vi "Update Expression.vi"(8 "error in (no error)":errorcluster, 10 "Expression":string, 11 "Cron in":refnum<class "Cron.lvclass">) -> (0 "error out":errorcluster, 1 "updated":bool, 3 "Cron out":refnum<class "Cron.lvclass">)   [LabVIEW 2013, in "openCron.lvlib" / "Cron.lvclass"]
uses:
  Cron.lvclass
  Cron.lvclass/Cron.ctl
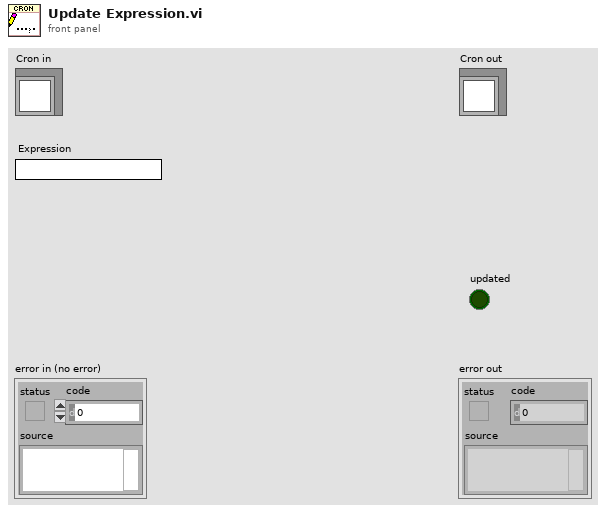
[diagram p1: front panel]
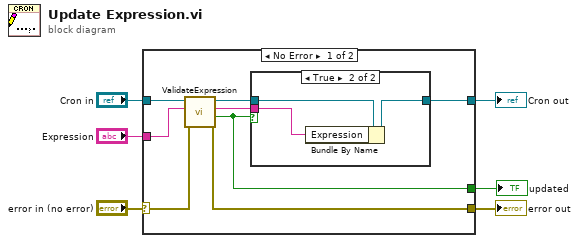
[diagram p0: block diagram]
diagram:
  n1 = case shown="No Error" "error in (no error)" {
    selector: "error in (no error)" -> [w8 w19]
    tunnel: [w7 w19] -> w5
    tunnel: [w11 w20] -> w3
    tunnel: "Cron in" -> [w14 w20]
    tunnel: "Expression" -> [w12 _]
    tunnel: [w9 _] -> w1
    frame No Error {
      n2 = call "ValidateExpression.vi"("error in (no error)"=w8, "Expression"=w12, "Cron in"=w14) -> ("error out"=w7:errorcluster, "valid?"=w9:bool, "Expression dup"=w10:string, "Cron out"=w13:refnum<class "Cron.lvclass">)  [unwired: 5 in]
      n3 = case shown="True" w9 {
        tunnel: w13 -> [w15 w18]
        tunnel: [w15 w17] -> w11
        tunnel: w10 -> [_ w16]
        frame False {
        }
        frame True {
          n4 = Bundle By Name(cluster=w18, "Expression"=w16) -> (w17:refnum<class "Cron.lvclass">)
        }
      }
    }
    frame Error {
    }
  }
  "error out" <- w5
  "Cron out" <- w3
  "updated" <- w1
